vi "_OpersList.vi"(8 "error in (no error)":errorcluster) -> (0 "error out":errorcluster, 2 "built-in VIFuncs":string[](array[string]), 3 "Array":refnum<vi>[](array[refnum]))   [LabVIEW 2017, in "tagdb-RefMgr Operations.lvlib"]
uses:
  tagdb-RefMgr Operations.lvlib
  VI/VI_ReinitializeAllToDefault.vi
  Control/Ctrls_SetValue.vi
  Control/Ctrls_ReinitializeToDefault.vi
  Control/Ctrls_Grayout.vi
  Control/Ctrls_Enable.vi
  Control/Ctrls_Disable.vi
  Menu/Menu_unCheck.vi
  Menu/Menu_ToggleEnable.vi
  Menu/Menu_ToggleCheck.vi
  Menu/Menu_ItemName.vi
  Menu/Menu_Enable.vi
  Menu/Menu_Disable.vi
  Menu/Menu_Check.vi
  VI/VI_ShowToolbar.vi
  VI/VI_ShowMenubar.vi
  VI/VI_ShowTitlebar.vi
  VI/VI_Minimizable.vi
  VI/VI_Resizable.vi
  VI/VI_Closeable.vi
  VI/VI_Frontmost.vi
  VI/VI_SetTitle.vi
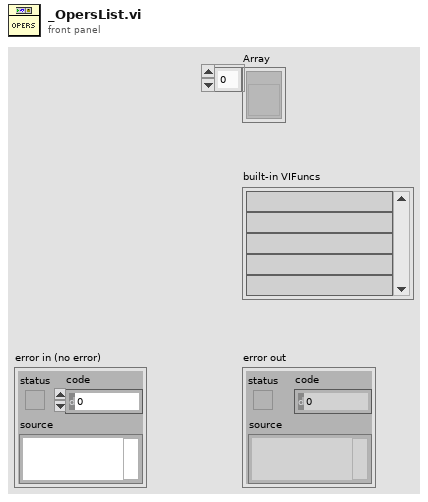
[diagram p1: front panel]
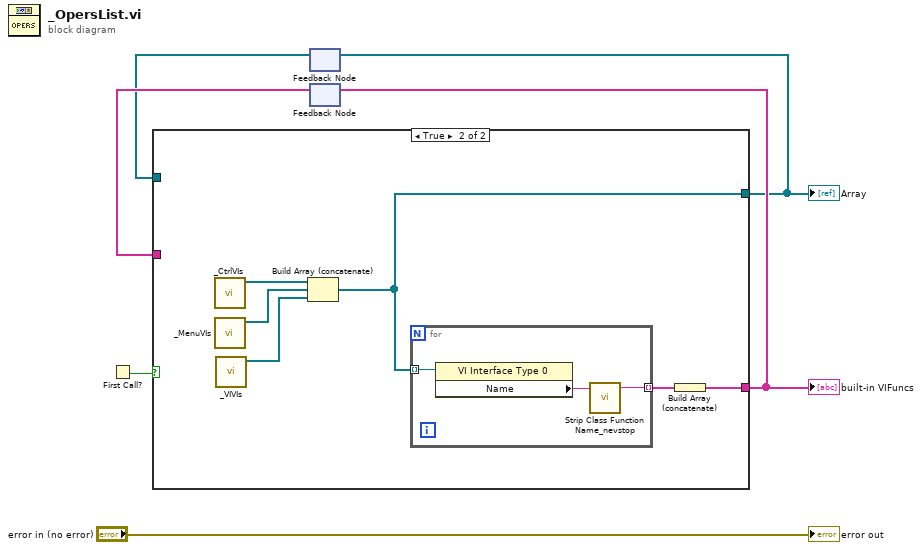
[diagram p0: block diagram]
diagram:
  n1 = First Call?() -> (First Call?: T/F=w5:bool)
  n2 = feedback #1() -> (w2:refnum<vi>[])  [unwired: 1 in]
  n3 = feedback #2() -> (w3:string[])  [unwired: 1 in]
  n4 = case shown="True" w5 {
    tunnel: [w8 w14] -> w4
    tunnel: [w7 w11] -> w1
    tunnel: w3 -> [w8 _]
    tunnel: w2 -> [w7 _]
    frame False {
    }
    frame True {
      n5 = call "_CtrlVIs.vi"() -> ("Array"=w12:refnum<vi>[])  [unwired: 11 in]
      n6 = call "_MenuVIs.vi"() -> ("VIs"=w10:refnum<vi>[])  [unwired: 11 in]
      n7 = call "_VIVIs.vi"() -> ("Array"=w9:refnum<vi>[])  [unwired: 11 in]
      n8 = Build Array (concatenate)(w12, w10, w9) -> (w11:refnum<vi>[])
      n9 = for {
        tunnel: w11 -> [w17] mode=indexing
        tunnel: [w15] -> w13 mode=indexing
        n10 = property class="VI Interface Type 0"(reference=w17) -> ("Name"=w16:string)  [unwired: 1 in, 2 out]
        n11 = call <userlib>:"Strip Class Function Name_nevstop.vi"("File Full Path Name"=w16) -> ("Function Name"=w15:string)  [unwired: 2 in, 2 out]
      }
      n12 = Build Array (concatenate)(w13) -> (w14:string[])
    }
  }
  "built-in VIFuncs" <- w4
  "Array" <- w1
  n13 = feedback-in #1(w1) -> ()
  n14 = feedback-in #2(w4) -> ()
  "error out" <- "error in (no error)"
